vi "_partDBEEPROMCmd_vcmd_vna_wmg.vi"(1 "input":string) -> (0 "output":string[][](array[string]))   [LabVIEW 2011]
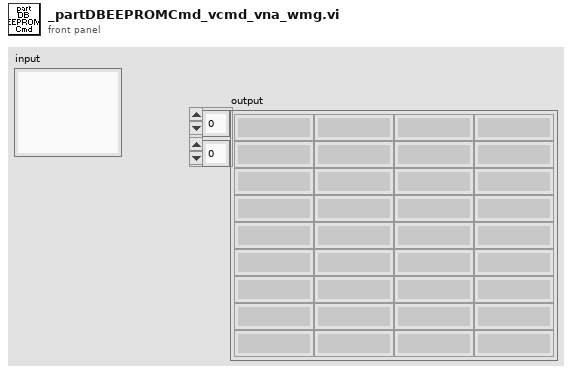
[diagram p1: front panel]
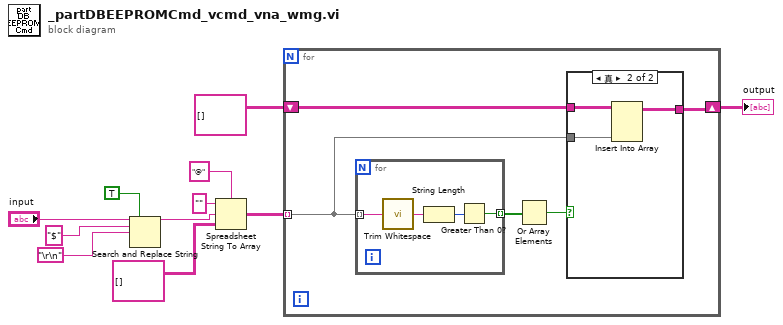
[diagram p0: block diagram]
diagram:
  n1 = Search and Replace String(replace all?=TRUE ("替换全部？(F)"), input string="input", search string="$", replace string="\r\n") -> (result string=w8:string)  [unwired: 4 in, 3 out]
  n2 = Spreadsheet String To Array(delimiter (Tab)="@" ("分隔符(Tab)"), format string="" ("格式字符串"), spreadsheet string=w8, array type (2D Dbl)=string[][] []) -> (array=w3:string[][])
  n3 = for {
    tunnel: w3 -> [w12] mode=indexing
    shift-right: [w13] -> w1
    shift-left: string[][] [] -> [w14]
    n4 = for {
      tunnel: w12 -> [w24] mode=indexing
      tunnel: [w21] -> w16 mode=indexing
      n5 = call <vilib>:"Trim Whitespace.vi"("string"=w24) -> ("trimmed string"=w23:string)  [unwired: 1 in]
      n6 = String Length(string=w23) -> (length=w22:i32)
      n7 = Greater Than 0?(x=w22) -> (x > 0?=w21:bool)
    }
    n8 = Or Array Elements(Boolean array=w16) -> (logical OR=w15:bool)
    n9 = case shown="真" w15 {
      tunnel: w14 -> [w17 w20]
      tunnel: [w17 w19] -> w13
      tunnel: w12 -> [_ w18]
      frame False {
      }
      frame True {
        n10 = Insert Into Array(array=w20, new element=w18) -> (w19:string[][])  [unwired: 2 in]
      }
    }
  }
  "output" <- w1
